vi "MODEL SELECTION.vi"(8 "error in (no error)":errorcluster, 11 "Plan List":string[](array[string])) -> (0 "error out 2":errorcluster, 3 "SCAN ADDON CODE RECIPE":string)   [LabVIEW 2017]
uses:
  Global/PLC_to_Auto.vi
panel:
  out "Scaned Code":string
  out "Stop scanner":bool
  in  "RECIPE SELECT":string(combo)
  in  "Cancel Button":bool
  in  "Save Button":bool
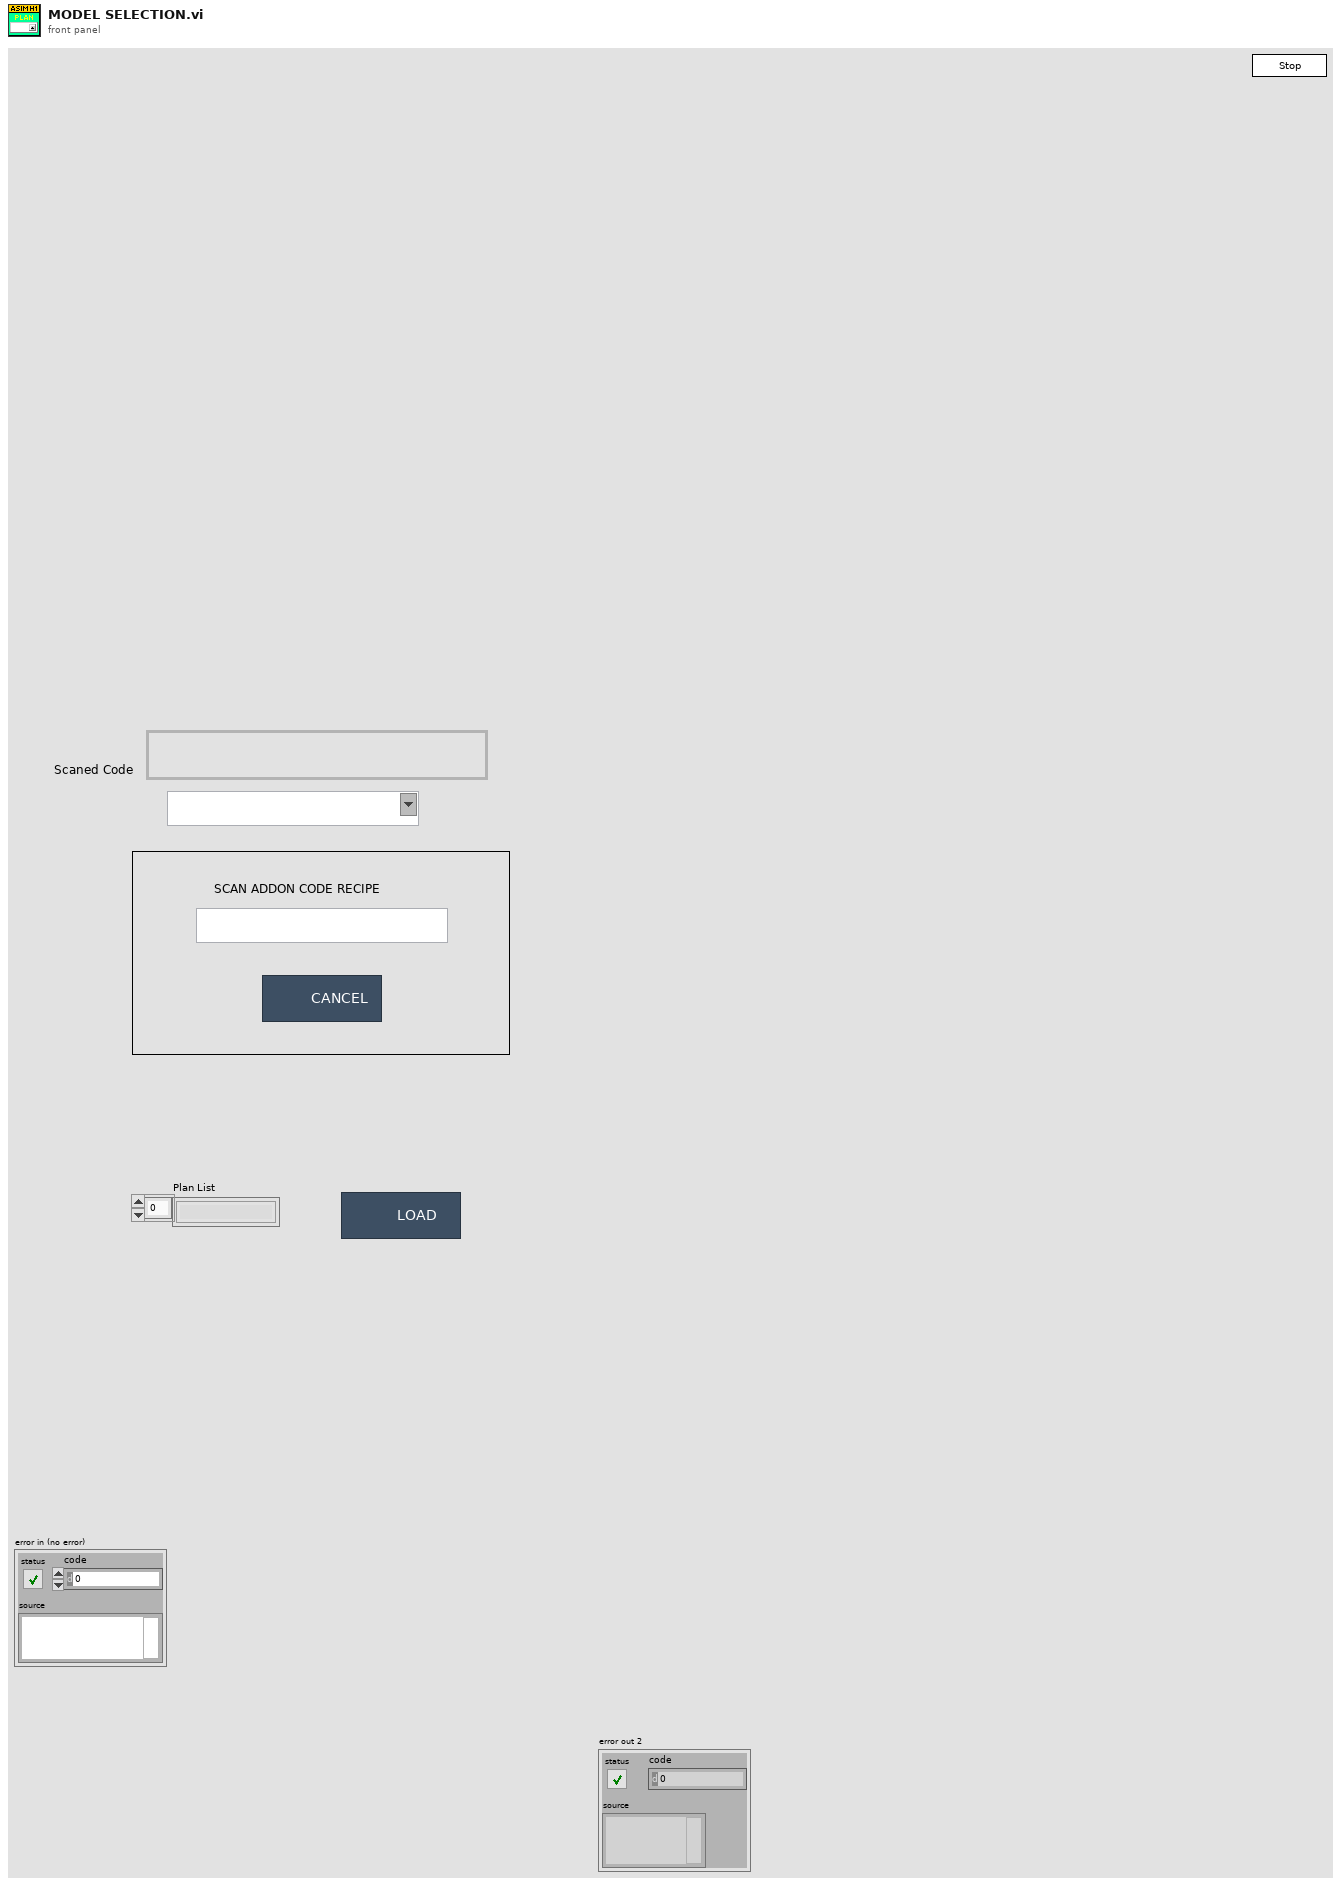
[diagram p1: front panel]
types:
  T1 = enum32{"invalid app kind", "Development System", "Run Time System", "Student Edition", "Embedded LabVIEW", "Evaluation", "Custom"}
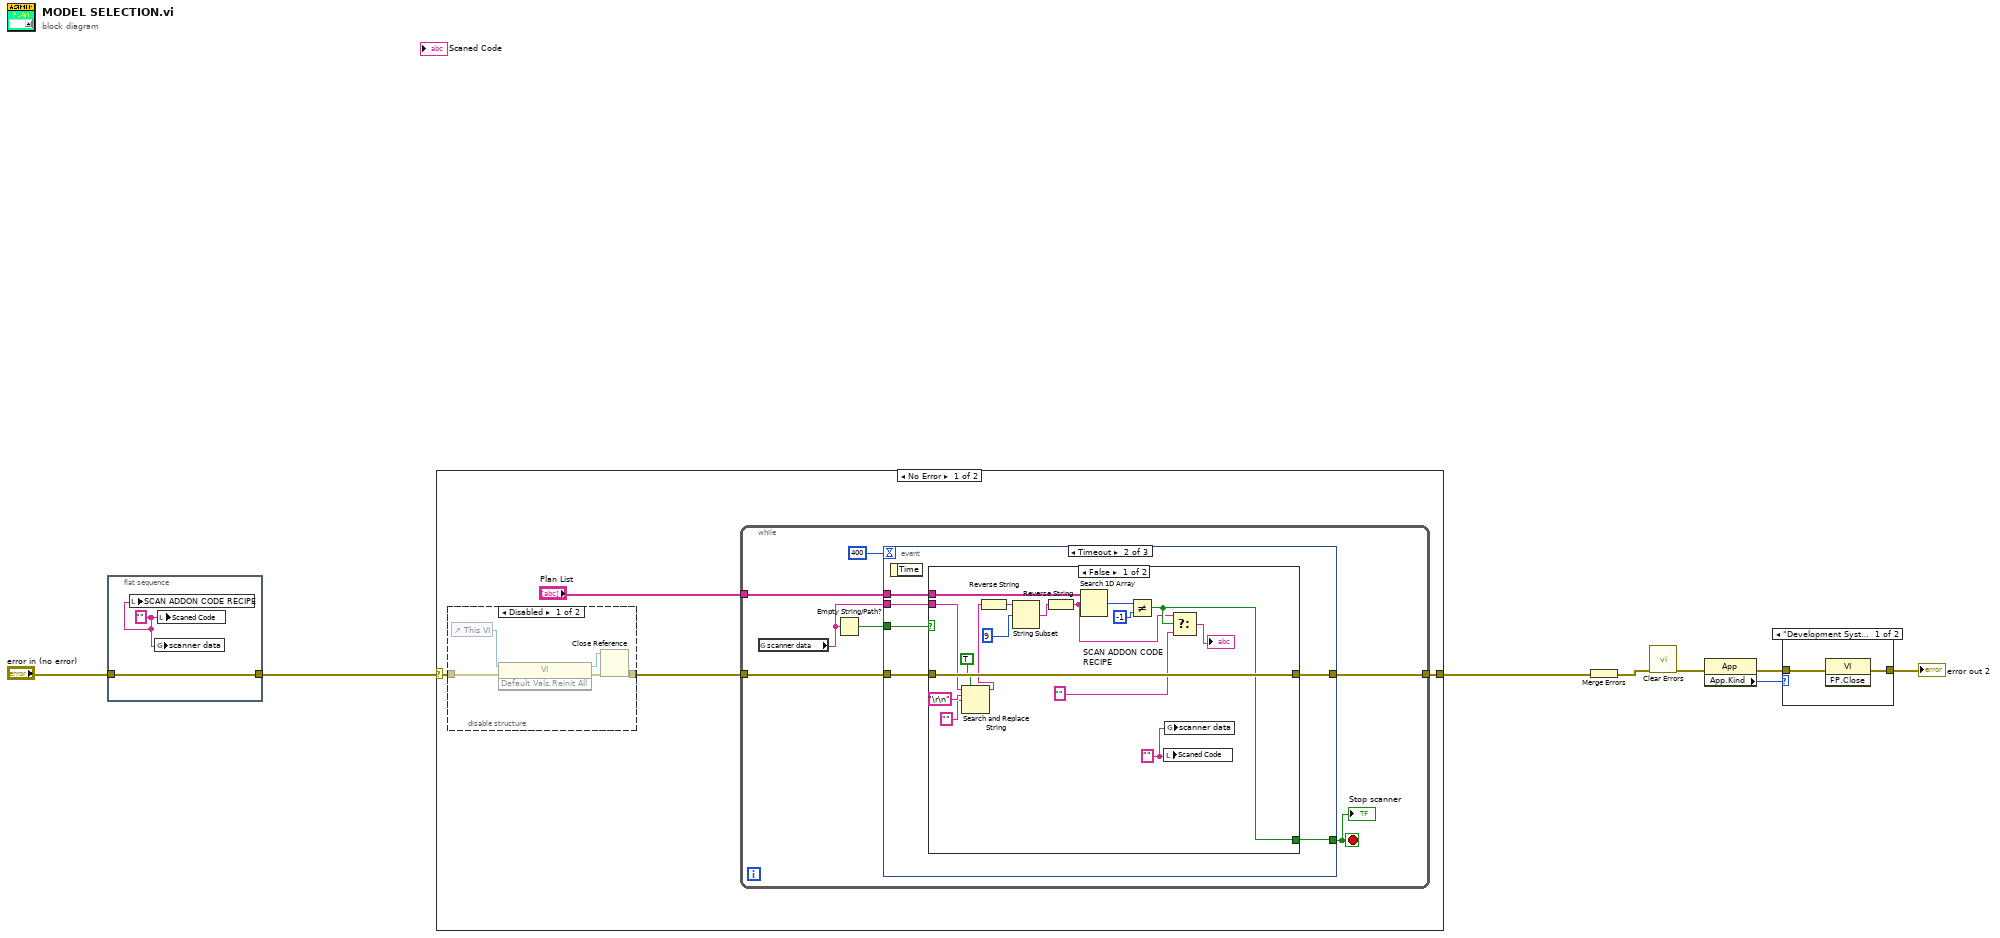
[diagram p0: block diagram]
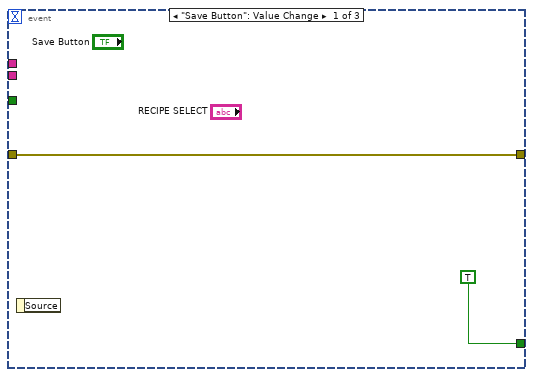
[diagram p3: hidden frame]
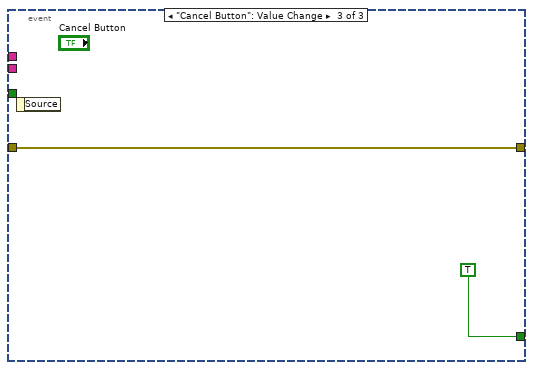
[diagram p5: hidden frame]
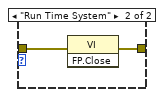
[diagram p7: hidden frame]
diagram:
  n1 = flat-sequence {
    tunnel: "error in (no error)" -> [w10]
    tunnel: [w10] -> w3
    frame #0 {
      w9 = ""
      n2 = local write "SCAN ADDON CODE RECIPE"(w9) -> ()
      n3 = global write "PLC_to_Auto.vi" "scanner data"(w9) -> ()
      n4 = local write "Scaned Code"(w9) -> ()
    }
  }
  n5 = case shown="No Error" w3 {
    selector: w3 -> [w13 w56]
    tunnel: [w14 w56] -> w8
    frame No Error {
      n6 = disable-structure shown="Disabled" {
        disable-tunnel: w13 -> [w18 w20]
        disable-tunnel: [w15 w20] -> w12
        frame Disabled {
          n7 = control-ref of="This VI"() -> (w19:refnum<vi>)
          n8 = invoke class="VI" method="Default Vals.Reinit All"(reference=w19, error in=w18) -> (reference out=w17:refnum<vi>, error out=w16:errorcluster)  [unwired: 1 in, 1 out]
          n9 = Close Reference(reference=w17, error in (no error)=w16) -> (error out=w15:errorcluster)
        }
        frame Enabled {
        }
      }
      n10 = while {
        tunnel: w12 -> [w26]
        tunnel: [w27] -> w14
        tunnel: "Plan List" -> [w24]
        stop <- w22 stop-if-true
        n11 = global read "PLC_to_Auto.vi" "scanner data"() -> (w21:string)
        n12 = Empty String/Path?(string/path=w21) -> (empty?=w23:bool)
        n13 = event shown="[1] Timeout" {
          selector: _ -> [_ _ _]
          dyn-events: _ -> [_ _ _]
          timeout: 400 -> [_ _ _]
          tunnel: [TRUE w30 TRUE] -> w22
          tunnel: [w28 w33 w54] -> w27
          tunnel: w26 -> [w28 w32 w54]
          tunnel: w24 -> [_ w35 _]
          tunnel: w23 -> [_ w34 _]
          tunnel: w21 -> [_ w31 _]
          event "Save Button": Value Change {
            n14 = event-data() -> ()  [unwired: 1 in, 1 out]
          }
          event Timeout {
            n15 = event-data() -> ()  [unwired: 1 in, 1 out]
            n16 = case shown="False" w34 {
              tunnel: w35 -> [w52 _]
              tunnel: [w51 w53] -> w33
              tunnel: w32 -> [w51 w53]
              tunnel: w31 -> [w39 _]
              tunnel: [w46 _] -> w30
              frame False {
                w36 = ""
                n17 = Search and Replace String(replace all?=TRUE, input string=w39, search string="\r\n", replace string="") -> (result string=w38:string)  [unwired: 4 in, 3 out]
                n18 = Reverse String(1:w38) -> (0:w50:string)
                n19 = String Subset(string=w50, offset (0)=9) -> (substring=w49:string)  [unwired: 1 in]
                n20 = Reverse String(1:w49) -> (0:w44:string)
                n21 = Search 1D Array(1D array=w52, element=w44) -> (index of element=w48:i32)  [unwired: 1 in]
                n22 = Not Equal?(x=w48, y=-1) -> (x != y?=w46:bool)
                n23 = local write "Scaned Code"(w36) -> ()
                n24 = global write "PLC_to_Auto.vi" "scanner data"(w36) -> ()
                n25 = Select(t=w44, s=w46, f="") -> (s? t:f=→"SCAN ADDON CODE RECIPE":string)
              }
              frame True {
              }
            }
          }
          event "Cancel Button": Value Change {
            n26 = event-data() -> ()  [unwired: 1 in, 1 out]
          }
        }
        "Stop scanner" <- w22
      }
    }
    frame Error {
    }
  }
  n27 = Merge Errors(w8) -> (w2:errorcluster)
  n28 = call <vilib>:"Clear Errors.vi"("error in (no error)"=w2) -> ("error out"=w1:errorcluster)  [unwired: 5 in, 1 out]
  n29 = property class="App"(error in=w1) -> (error out=w6:errorcluster, "App.Kind"=w5:T1)  [unwired: 1 in, 1 out]
  n30 = case shown="\"Development System\", Default" w5 {
    tunnel: [w57 w60] -> w7
    tunnel: w6 -> [w58 w59]
    frame "Development System", Default {
      n31 = invoke class="VI" method="FP.Close"(error in=w58) -> (error out=w57:errorcluster)  [unwired: 2 in, 2 out]
    }
    frame "Run Time System" {
      n32 = invoke class="VI" method="FP.Close"(error in=w59) -> (error out=w60:errorcluster)  [unwired: 2 in, 2 out]
    }
  }
  "error out 2" <- w7
